vi "Write ROI.vi"(8 "error in (no error)":errorcluster, 10 "ROI":T1, 11 "Camera Data in":refnum<class "Camera Data.lvclass">) -> (0 "error out":errorcluster, 3 "Camera Data out":refnum<class "Camera Data.lvclass">)   [LabVIEW 2022 SP3, in "Camera Data.lvclass"]
uses:
  Camera Data.lvclass
  Camera Data.lvclass/Camera Data.ctl
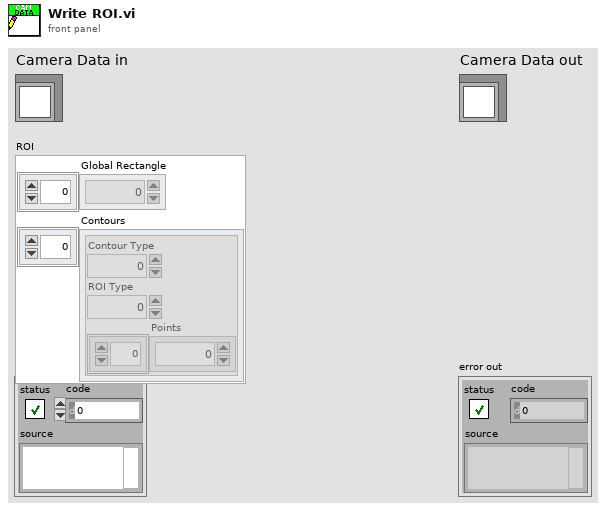
[diagram p1: front panel]
types:
  T1 = cluster{"Global Rectangle":i32[], "Contours":cluster{"Contour Type":u32, "ROI Type":u32, "Points":i32[]}[]}
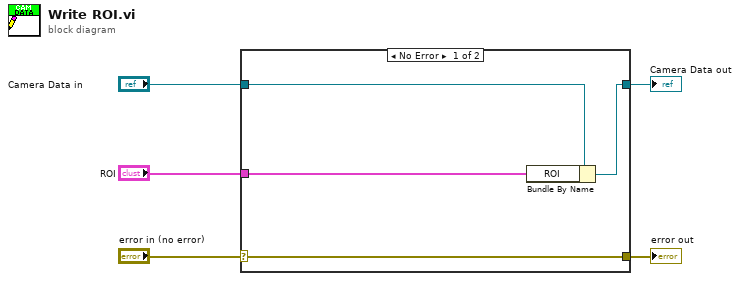
[diagram p0: block diagram]
diagram:
  n1 = case shown="No Error" "error in (no error)" {
    selector: "error in (no error)" -> [w9 w10]
    tunnel: [w9 w10] -> w4
    tunnel: [w7 w11] -> w2
    tunnel: "Camera Data in" -> [w8 w11]
    tunnel: "ROI" -> [w6 _]
    frame No Error {
      n2 = Bundle By Name(cluster=w8, "ROI"=w6) -> (w7:refnum<class "Camera Data.lvclass">)
    }
    frame Error {
    }
  }
  "error out" <- w4
  "Camera Data out" <- w2
